vi "DSP Loop.vi"(7 "数据通知器处理":refnum<notifier>, 8 "error in (no error)":errorcluster caption="错误输入（无错误）", 9 "数据通知器原始":refnum<notifier>, 10 "DSP":refnum<queue>, 11 "Director":refnum<queue>) -> (0 "error out":errorcluster caption="错误输出")   [LabVIEW 2015, in "Digital Signal Processing.lvlib"]
doc: "该消息循环负责处理硬件数据采集的相关消息。"
uses:
  Digital Signal Processing.lvlib
  support/Message Queue/Message Cluster.ctl
  Support/DSP State.ctl
  Support/DSP Configuration.ctl
  <vilib>/Analysis/3filter.llb/Filter Passband Type.ctl
  <vilib>/Analysis/4window.llb/windowTd.ctl
  Support/DSP Parameter.ctl
  support/Message Queue/Enqueue Message (Single).vi
  <vilib>/Utility/error.llb/Error Cluster From Error Code.vi
  <vilib>/ErrorRing/Error Ring.xnode
  support/Message Queue/Message Queue.lvlib
  DAQ/DAQ.lvlib
  <vilib>/Analysis/NI_AALBase.lvlib
  <vilib>/Analysis/NI_AALPro.lvlib
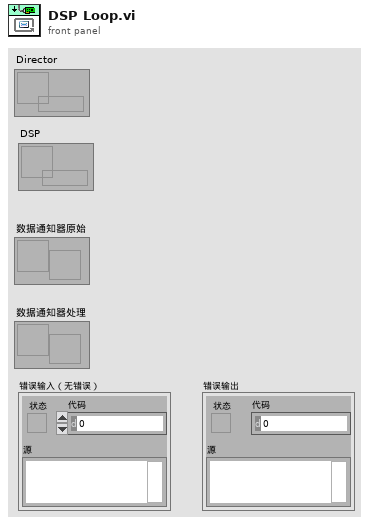
[diagram p1: front panel]
types:
  T1 = typedef "Digital Signal Processing.lvlib/DSP Parameter.ctl" = cluster{"RF":cluster{"filter structure":enum32{"IIR 2nd Order", "IIR 4th Order"}, "Reverse Coefficients":dbl[], "Forward Coefficients":dbl[]}, "IIR Filter Cluster":cluster{"filter structure":enum32{"IIR 2nd Order", "IIR 4th Order"}, "Reverse Coefficients":dbl[], "Forward Coefficients":dbl[]}, "Noise Signal":dbl[], "SPAN":i32, "Logarithmic Base":dbl}
  T2 = typedef "Digital Signal Processing.lvlib/DSP Configuration.ctl" = cluster{"Sampling Frequency":dbl, "filter type":T3, "RF Filter Low Frequency":dbl, "RF Filter High Frequency":dbl, "RF Filter Taps":i32, "window":T4, "RF window parameter":dbl, "filter type 2":T3, "Demodulated Filter Low Frequency":dbl, "Demodulated Filter HighFrequency":dbl, "Demodulated Filter Order":i32, "SPAN":i32, "Logarithmic Base":dbl, "Noise path":string, "Work position parameter":i32[]}
  T3 = typedef "NI_AALBase.lvlib/Filter Passband Type.ctl" = enum32{"Lowpass", "Highpass", "Bandpass", "Bandstop"}
  T4 = typedef "NI_AALPro.lvlib/windowTd.ctl" = u32
  T5 = typedef "Digital Signal Processing.lvlib/DSP State.ctl" = enum16{"Idle", "Processing"}
  T6 = cluster{"filter structure":enum32{"IIR 2nd Order", "IIR 4th Order"}, "Reverse Coefficients":dbl[], "Forward Coefficients":dbl[]}
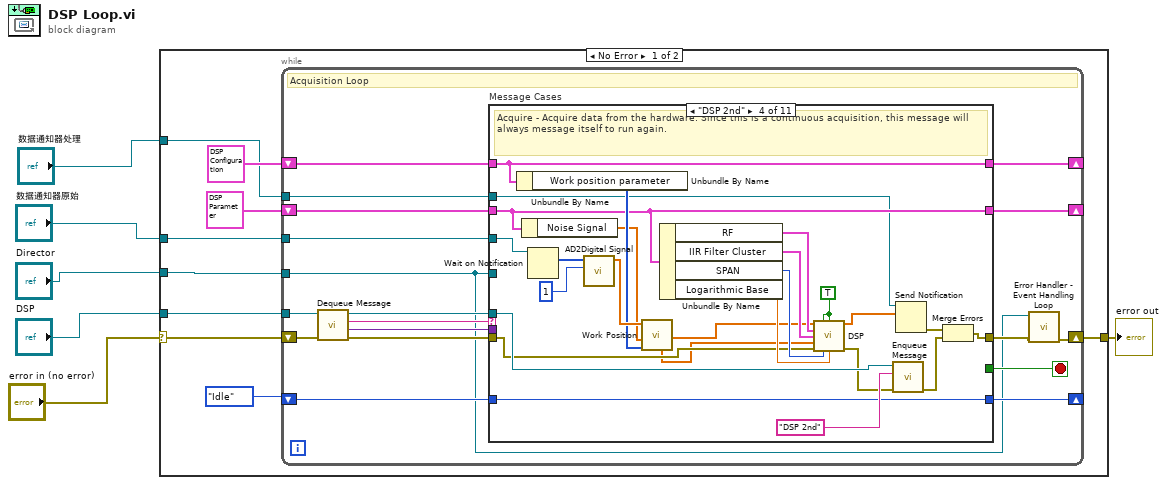
[diagram p0: block diagram]
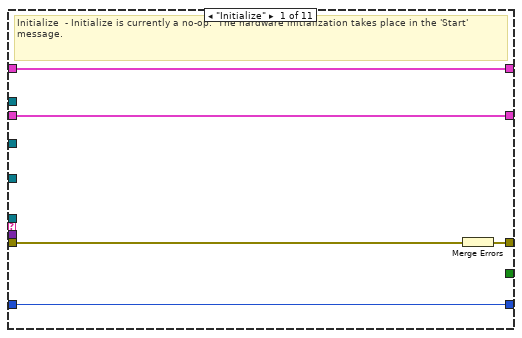
[diagram p2: hidden frame]
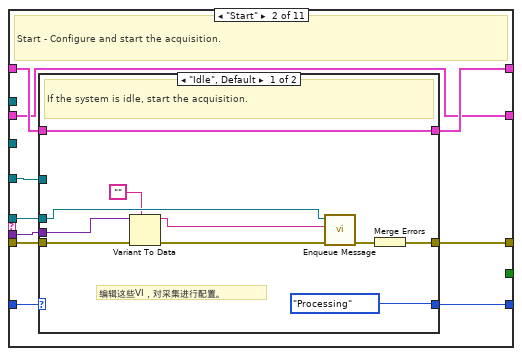
[diagram p3: hidden frame]
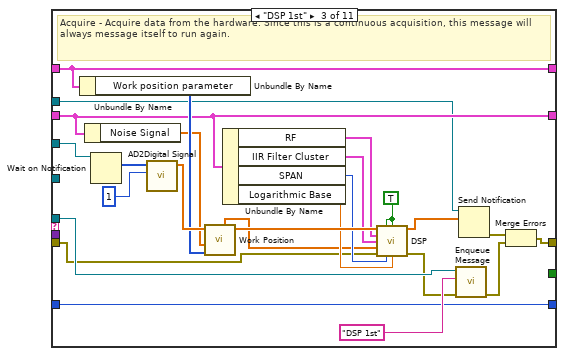
[diagram p5: hidden frame]
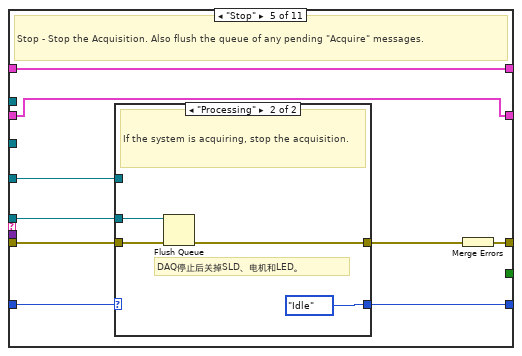
[diagram p6: hidden frame]
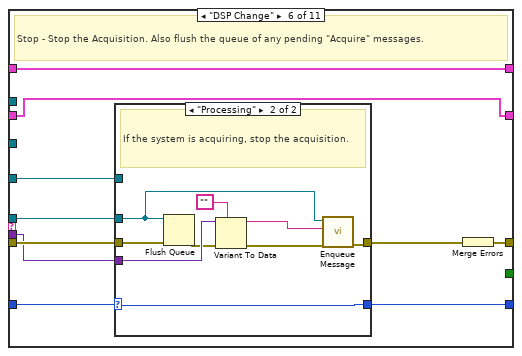
[diagram p8: hidden frame]
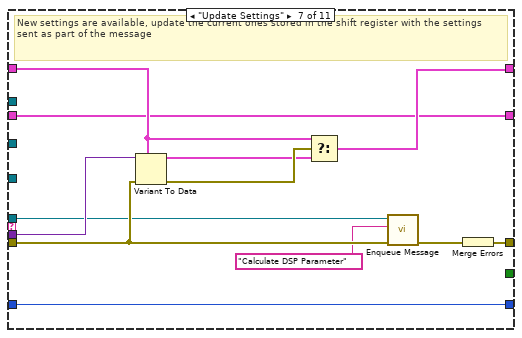
[diagram p10: hidden frame]
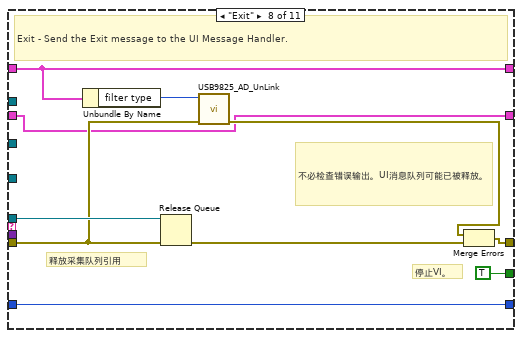
[diagram p11: hidden frame]
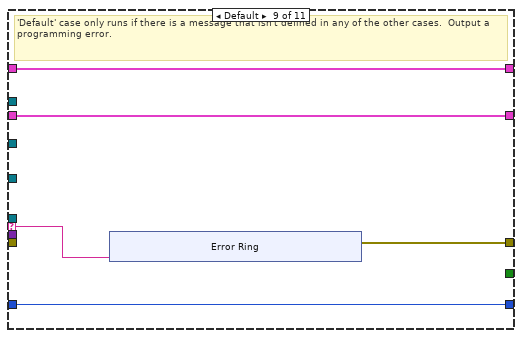
[diagram p12: hidden frame]
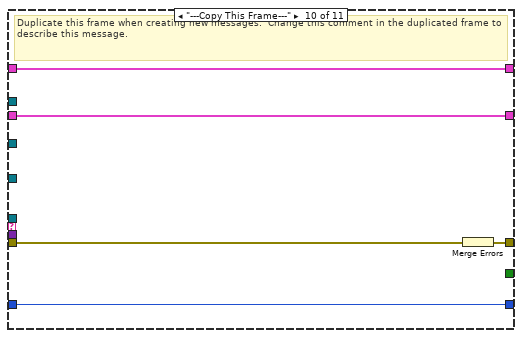
[diagram p13: hidden frame]
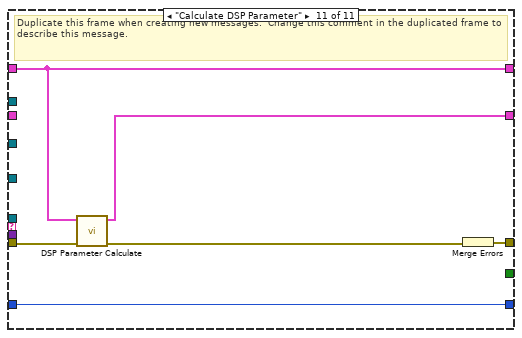
[diagram p14: hidden frame]
diagram:
  n1 = case shown="No Error" "error in (no error)" {
    selector: "error in (no error)" -> [w14 w193]
    tunnel: [w15 w193] -> w6
    tunnel: "数据通知器原始" -> [w13 _]
    tunnel: "DSP" -> [w12 _]
    tunnel: "Director" -> [w11 _]
    tunnel: "数据通知器处理" -> [w7 _]
    frame No Error {
      n2 = while {
        tunnel: w12 -> [w25]
        shift-right: [w32] -> _
        shift-left: T2 {"Sampling Frequency"=0.0, "filter type"=enum."Lowpass", "RF Filter Low Frequency"=0.0, "RF Filter High Frequency"=0.0, "RF Filter Taps"=0, "window"=0, "RF window parameter"=nan, "filter type 2"=enum."Lowpass", "Demodulated Filter Low Frequency"=0.0, "Demodulated Filter HighFrequency"=0.0, "Demodulated Filter Order"=0, "SPAN"=0, "Logarithmic Base"=0.0, "Noise path"="", "Work position parameter"=[]} ("DSP Configuration") -> [w33]
        shift-right: [w22] -> w15
        shift-left: w14 -> [w30]
        tunnel: w11 -> [w20]
        shift-right: [w23] -> _
        shift-left: DSP_State."Idle" ("State") -> [w24]
        tunnel: w13 -> [w19]
        shift-right: [w17] -> _
        shift-left: T1 {"RF"={"filter structure"=enum."IIR 2nd Order", "Reverse Coefficients"=[], "Forward Coefficients"=[]}, "IIR Filter Cluster"={"filter structure"=enum."IIR 2nd Order", "Reverse Coefficients"=[], "Forward Coefficients"=[]}, "Noise Signal"=[], "SPAN"=0, "Logarithmic Base"=0.0} ("DSP Parameter") -> [w18]
        tunnel: w7 -> [w16]
        stop <- w31 stop-if-true
        # "Acquisition Loop"
        n3 = call "Dequeue Message.vi"("error in (no error)"=w30, "消息队列"=w25) -> ("error out"=w29:cluster{"状态":bool, "代码":i32, "源":string}, "消息数据"=w27:variant, "消息"=w28:string, "消息队列副本"=w26:refnum<queue>)  [unwired: 6 in]
        n4 = case "Message Cases" shown="\"DSP 2nd\"" w28 {
          selector: w28 -> [_ _ _ _ _ _ _ _ w173 _ _]
          tunnel: w26 -> [_ w45 w84 w109 w117 w133 w149 w166 _ _ _]
          tunnel: w29 -> [w36 w46 w66 w93 w119 w135 w151 w162 _ w186 w190]
          tunnel: [w38 w48 w86 w111 w120 w136 w159 w168 w172 w184 w192] -> w21
          tunnel: w33 -> [w35 w47 w76 w101 w118 w134 w155 w164 w174 w185 w188]
          tunnel: [w35 w44 w76 w101 w118 w134 w154 w164 w174 w185 w188] -> w32
          tunnel: [_ _ _ _ _ _ _ TRUE _ _ _] -> w31
          tunnel: w27 -> [_ w39 _ _ _ w127 w158 _ _ _ _]
          tunnel: w20 -> [_ w41 _ _ w116 w132 _ _ _ _ _]
          tunnel: w24 -> [w37 w43 w82 w107 w115 w131 w153 w165 w171 w183 w191]
          tunnel: [w37 w42 w82 w107 w114 w130 w153 w165 w171 w183 w191] -> w23
          tunnel: w19 -> [_ _ w80 w105 _ _ _ _ _ _ _]
          tunnel: w18 -> [w34 w40 w72 w98 w112 w128 w152 w160 w170 w182 _]
          tunnel: [w34 w40 w72 w98 w112 w128 w152 w160 w170 w182 w187] -> w17
          tunnel: w16 -> [_ _ w64 w91 _ _ _ _ _ _ _]
          frame "Initialize" {
            # "Initialize  - Initialize is currently a no-op.  The hardware initialization takes place in the 'Start' message."
            n5 = Merge Errors(w36) -> (w38:errorcluster)
          }
          frame "Start" {
            # "Start - Configure and start the acquisition."
            n6 = case shown="\"Idle\", Default" w43 {
              selector: w43 -> [_ w59]
              tunnel: [w58 w61] -> w48
              tunnel: w47 -> [w55 w60]
              tunnel: w46 -> [w53 w61]
              tunnel: w45 -> [w56 _]
              tunnel: [w55 w60] -> w44
              tunnel: [DSP_State."Processing" ("State") w59] -> w42
              tunnel: w41 -> [_ _]
              tunnel: w39 -> [w51 _]
              frame "Idle", Default {
                # "编辑这些VI，对采集进行配置。"
                # "If the system is idle, start the acquisition."
                n7 = Variant To Data(error in=w53, type="", Variant=w51) -> (data=w49:string, error out=w52:errorcluster)
                n8 = call-poly "Enqueue Message.vi"("error in (no error)"=w52, "消息"=w49, "消息队列"=w56) -> ("error out"=w57:cluster{"状态":bool, "代码":i32, "源":string})  [unwired: 7 in, 1 out]
                n9 = Merge Errors(w57) -> (w58:errorcluster)
              }
              frame "Processing" {
                # "The system is already acquiring. Ignore the \"Start\" message."
              }
            }
          }
          frame "DSP 1st" {
            w62 = TRUE ("Minus Noise(F : Don't)")
            # "Acquire - Acquire data from the hardware. Since this is a continuous acquisition, this message will always message itself to run again."
            n10 = Unbundle By Name(w76) -> ("Work position parameter"=w75:i32[])
            n11 = Unbundle By Name(w72) -> ("Noise Signal"=w74:dbl[])
            n12 = Wait on Notification(notifier=w80) -> (notification=w79:i16[])  [unwired: 3 in, 3 out]
            n13 = call "AD2Digital Signal.vi"("通道数"=1, "AD"=w79) -> ("CH1"=w77:dbl[])  [unwired: 8 in, 1 out]
            n14 = call "Work Position.vi"("Work position parameter"=w75, "Noise"=w74, "S"=w77) -> ("S_1st_part"=w73:dbl[], "Noise_1st_part"=w67:dbl[])  [unwired: 3 in, 4 out]
            n15 = Unbundle By Name(w72) -> ("RF"=w71:T6, "IIR Filter Cluster"=w70:T6, "SPAN"=w69:i32, "Logarithmic Base"=w68:dbl)
            n16 = call "DSP.vi"("Input Signal"=w73, "Smooth(F : Don't)"=w62, "Minus Noise(F : Don't)"=w62, "RF"=w71, "IIR Filter Cluster"=w70, "Noise Signal"=w67, "error in (no error)"=w66, "SPAN"=w69, "Logarithmic Base"=w68) -> ("DSP signal"=w65:dbl[], "error out"=w63:errorcluster)  [unwired: 5 in]
            n17 = call-poly "Enqueue Message.vi"("error in (no error)"=w63, "消息"="DSP 1st" ("Message"), "消息队列"=w84) -> ("error out"=w85:cluster{"状态":bool, "代码":i32, "源":string})  [unwired: 7 in, 1 out]
            n18 = Send Notification(notification=w65, notifier=w64) -> (error out=w81:errorcluster)  [unwired: 1 in, 1 out]
            n19 = Merge Errors(w81, w85) -> (w86:errorcluster)
          }
          frame "DSP 2nd" {
            w87 = TRUE ("Minus Noise(F : Don't)")
            # "Acquire - Acquire data from the hardware. Since this is a continuous acquisition, this message will always message itself to run again."
            n20 = Unbundle By Name(w101) -> ("Work position parameter"=w100:i32[])
            n21 = Unbundle By Name(w98) -> ("Noise Signal"=w99:dbl[])
            n22 = Wait on Notification(notifier=w105) -> (notification=w104:i16[])  [unwired: 3 in, 3 out]
            n23 = call "AD2Digital Signal.vi"("通道数"=1, "AD"=w104) -> ("CH1"=w102:dbl[])  [unwired: 8 in, 1 out]
            n24 = call "Work Position.vi"("Work position parameter"=w100, "Noise"=w99, "S"=w102) -> ("S_2nd_part"=w90:dbl[], "Noise_2nd_part"=w89:dbl[])  [unwired: 3 in, 4 out]
            n25 = Unbundle By Name(w98) -> ("RF"=w97:T6, "IIR Filter Cluster"=w96:T6, "SPAN"=w95:i32, "Logarithmic Base"=w94:dbl)
            n26 = call "DSP.vi"("Input Signal"=w90, "Smooth(F : Don't)"=w87, "Minus Noise(F : Don't)"=w87, "RF"=w97, "IIR Filter Cluster"=w96, "Noise Signal"=w89, "error in (no error)"=w93, "SPAN"=w95, "Logarithmic Base"=w94) -> ("DSP signal"=w92:dbl[], "error out"=w88:errorcluster)  [unwired: 5 in]
            n27 = call-poly "Enqueue Message.vi"("error in (no error)"=w88, "消息"="DSP 2nd" ("Message"), "消息队列"=w109) -> ("error out"=w110:cluster{"状态":bool, "代码":i32, "源":string})  [unwired: 7 in, 1 out]
            n28 = Send Notification(notification=w92, notifier=w91) -> (error out=w106:errorcluster)  [unwired: 1 in, 1 out]
            n29 = Merge Errors(w106, w110) -> (w111:errorcluster)
          }
          frame "Stop" {
            # "Stop - Stop the Acquisition. Also flush the queue of any pending \"Acquire\" messages."
            n30 = case shown="\"Processing\"" w115 {
              selector: w115 -> [w122 _]
              tunnel: w119 -> [w121 w126]
              tunnel: w117 -> [_ w125]
              tunnel: w116 -> [_ _]
              tunnel: [w122 DSP_State."Idle" ("State")] -> w114
              tunnel: [w121 w124] -> w113
              frame "Idle", Default {
                # "The system is already idle. Ignore the \"Stop\" message."
              }
              frame "Processing" {
                # "DAQ停止后关掉SLD、电机和LED。"
                # "If the system is acquiring, stop the acquisition."
                n31 = Flush Queue(queue=w125, error in (no error)=w126) -> (error out=w124:errorcluster)  [unwired: 2 out]
              }
            }
            n32 = Merge Errors(w113) -> (w120:errorcluster)
          }
          frame "DSP Change" {
            # "Stop - Stop the Acquisition. Also flush the queue of any pending \"Acquire\" messages."
            n33 = case shown="\"Processing\"" w131 {
              selector: w131 -> [w138 w146]
              tunnel: w135 -> [w137 w147]
              tunnel: w133 -> [_ w144]
              tunnel: w132 -> [_ _]
              tunnel: [w138 w146] -> w130
              tunnel: [w137 w145] -> w129
              tunnel: w127 -> [_ w143]
              frame "Idle", Default {
                # "The system is already idle. Ignore the \"Stop\" message."
              }
              frame "Processing" {
                # "If the system is acquiring, stop the acquisition."
                n34 = Flush Queue(queue=w144, error in (no error)=w147) -> (error out=w141:errorcluster)  [unwired: 2 out]
                n35 = Variant To Data(error in=w141, type="", Variant=w143) -> (data=w139:string, error out=w140:errorcluster)
                n36 = call-poly "Enqueue Message.vi"("error in (no error)"=w140, "消息"=w139, "消息队列"=w144) -> ("error out"=w145:cluster{"状态":bool, "代码":i32, "源":string})  [unwired: 7 in, 1 out]
              }
            }
            n37 = Merge Errors(w129) -> (w136:errorcluster)
          }
          frame "Update Settings" {
            # "New settings are available, update the current ones stored in the shift register with the settings sent as part of the message"
            n38 = Variant To Data(error in=w151, type=w155, Variant=w158) -> (data=w156:T2, error out=w157:errorcluster)
            n39 = Select(t=w155, s=w157, f=w156) -> (s? t:f=w154:T2)
            n40 = call-poly "Enqueue Message.vi"("error in (no error)"=w151, "消息"="Calculate DSP Parameter", "消息队列"=w149) -> ("error out"=w150:cluster{"状态":bool, "代码":i32, "源":string})  [unwired: 7 in, 1 out]
            n41 = Merge Errors(w150) -> (w159:errorcluster)
          }
          frame "Exit" {
            # "不必检查错误输出。UI消息队列可能已被释放。"
            # "释放采集队列引用"
            # "停止VI。"
            # "Exit - Send the Exit message to the UI Message Handler."
            n42 = Unbundle By Name(w164) -> ("filter type"=w163:T3)
            n43 = Release Queue(queue=w166, error in (no error)=w162) -> (error out=w167:errorcluster)  [unwired: 1 in, 2 out]
            n44 = call "USB9825_AD_UnLink.vi"("Error In"=w162, "hDevice"=w163) -> ("Error Out"=w161:errorcluster)  [unwired: 9 in]
            n45 = Merge Errors(w161, w167) -> (w168:errorcluster)
          }
          frame Default {
            # "'Default' case only runs if there is a message that isn't defined in any of the other cases.  Output a programming error."
            n46 = xnode "Error Ring"("parameter 0"=w173) -> ("error out"=w172:errorcluster)
          }
          frame "---Copy This Frame---" {
            # "Duplicate this frame when creating new messages.  Change this comment in the duplicated frame to describe this message."
            n47 = Merge Errors(w186) -> (w184:errorcluster)
          }
          frame "Calculate DSP Parameter" {
            # "Duplicate this frame when creating new messages.  Change this comment in the duplicated frame to describe this message."
            n48 = call "DSP Parameter Calculate.vi"("error in (no error)"=w190, "DSP Configuration"=w188) -> ("error out"=w189:errorcluster, "DSP Parameter"=w187:T1)  [unwired: 8 in]
            n49 = Merge Errors(w189) -> (w192:errorcluster)
          }
        }
        n50 = call "Error Handler - Event Handling Loop.vi"("error in (no error)"=w21, "消息队列"=w20) -> ("错误输入副本"=w22:cluster{"状态":bool, "代码":i32, "源":string})  [unwired: 8 in, 1 out]
      }
    }
    frame Error {
    }
  }
  "error out" <- w6
